vi "writeToXML.vi"(8 "error in (no error)":errorcluster, 10 "ClassLabel":string, 11 "Planet in":refnum<class "Planet.lvclass">) -> (0 "error out":errorcluster, 2 "XMLout":string, 3 "Planet out":refnum<class "Planet.lvclass">)   [LabVIEW 2022 SP3, in "TCSDataDefinitions.lvlib" / "TCSCommand.lvlib" / "TargetConfiguration.lvlib" / "Target.lvlib" / "Planet.lvclass"]
uses:
  Planet.lvclass
  Planet.lvclass/Planet.ctl
  Target/Target.lvclass
  <userlib>/Common/XML/XMLGenerator/XMLGenerator.lvclass
  <userlib>/Common/XML/XMLAttributeGenerator/XMLAttributeGenerator.lvclass
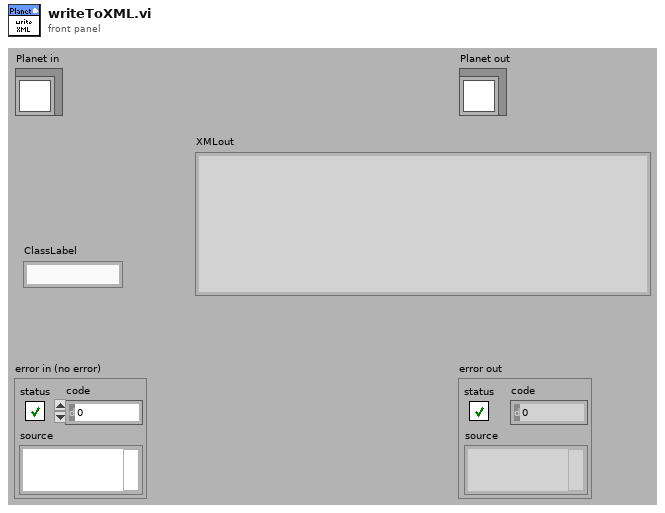
[diagram p1: front panel]
types:
  T1 = typedef "TCSDataDefinitions.lvlib/TCSCommand.lvlib/TargetConfiguration.lvlib/Target.lvlib/PlanetNameValues.ctl" = enum16{"Mercury", "Venus", "Moon", "Mars", "Jupiter", "Saturn", "Uranus", "Neptune", "Pluto"}
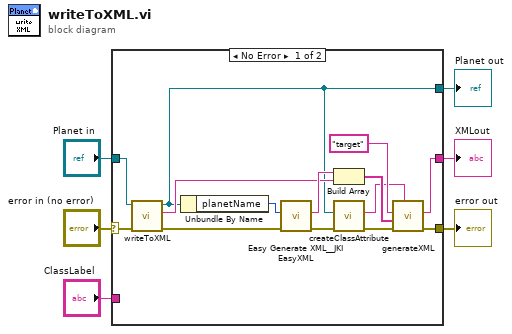
[diagram p0: block diagram]
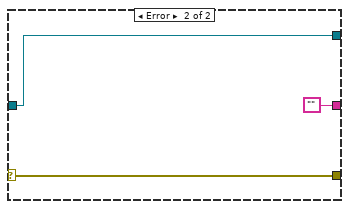
[diagram p2: hidden frame]
diagram:
  n1 = case shown="No Error" "error in (no error)" {
    selector: "error in (no error)" -> [w15 w23]
    tunnel: [w14 w23] -> w5
    tunnel: [w10 w22] -> w3
    tunnel: "Planet in" -> [w20 w22]
    tunnel: [w12 ""] -> w2
    tunnel: "ClassLabel" -> [_ _]
    frame No Error {
      n2 = call-parent "writeToXML.vi"("error in (no error)"=w15, "Target in"=w20) -> ("error out"=w16:errorcluster, "XML out"=w17:string, "Target out"=w10:refnum<class "Planet.lvclass">)  [unwired: 7 in]
      n3 = Unbundle By Name(w10) -> ("planetName"=w19:T1)
      n4 = call <vilib>:"Easy Generate XML__JKI EasyXML.vi"("error in (no error)"=w16, "LabVIEW Data"=w19) -> ("error out"=w9:errorcluster, "XML String"=w18:string)  [unwired: 8 in]
      n5 = Build Array(w18, w17) -> (w13:string[])
      n6 = call <userlib>:"createClassAttribute.vi"("error in (no error)"=w9, "LVClass In"=w10) -> ("error out"=w8:errorcluster, "AttributeString"=w7:string)  [unwired: 7 in, 1 out]
      n7 = call <userlib>:"generateXML.vi"("attributeString"=w7, "error in"=w8, "childrenXML"=w13, "elementName"="target" ("Class Label")) -> ("error out"=w14:errorcluster, "XML out"=w12:string)  [unwired: 5 in, 1 out]
    }
    frame Error {
    }
  }
  "error out" <- w5
  "Planet out" <- w3
  "XMLout" <- w2
